vi "Close Spreadsheet.vi"(8 "error in (no error)":errorcluster, 11 "Excel Legacy in":refnum<class "Excel Legacy.lvclass">) -> (0 "error out":errorcluster, 3 "Excel Legacy out":refnum<class "Excel Legacy.lvclass">)   [LabVIEW 2013, in "Excel Legacy.lvclass"]
uses:
  Excel Legacy.lvclass
  Spreadsheet.lvclass
  C:/PhaeronGit/LVNPOI/Resources/NPOI 2.1.1 dotnet2/NPOI.dll
  Resources/NPOI 2.1.1 dotnet2/NPOI.dll
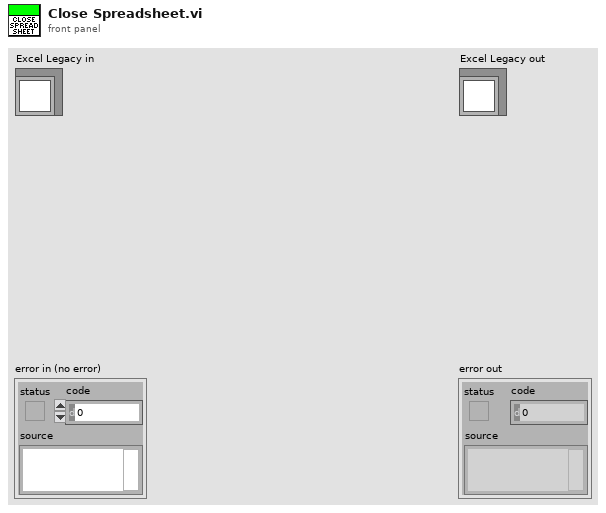
[diagram p1: front panel]
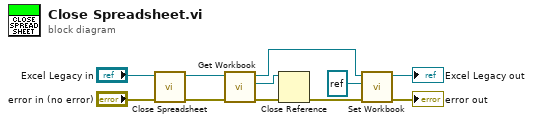
[diagram p0: block diagram]
diagram:
  n1 = call-parent "Close Spreadsheet.vi"("error in (no error)"="error in (no error)", "Spreadsheet in"="Excel Legacy in") -> ("error out"=w8:errorcluster, "Spreadsheet out"=w9:refnum<class "Excel Legacy.lvclass">)  [unwired: 8 in]
  n2 = call-dynamic "Get Workbook.vi"("error in (no error)"=w8, "Excel Legacy in"=w9) -> ("error out"=w3:errorcluster, "Workbook"=w1:refnum<k24>, "Excel Legacy out"=w6:refnum<class "Excel Legacy.lvclass">)  [unwired: 7 in]
  n3 = Close Reference(reference=w1, error in (no error)=w3) -> (error out=w2:errorcluster)
  n4 = call-dynamic "Set Workbook.vi"("error in (no error)"=w2, "Workbook"=refnum<k24> refnum, "Excel Legacy in"=w6) -> ("error out"=→"error out":errorcluster, "Excel Legacy out"=→"Excel Legacy out":refnum<class "Excel Legacy.lvclass">)  [unwired: 7 in]
